vi "Trans-RT.vi"() -> ()   [LabVIEW 2016]
uses:
  <vilib>/rvi/interface/nirviOpenFPGA/nirviOpenFPGA.xnode
  <vilib>/rvi/interface/nirviReadWriteControl/nirviReadWriteControl.xnode
  <vilib>/functionblocks/FB Core/FB Core.xnode
  <vilib>/functionblocks/Control/PID/PID.vi
  <vilib>/functionblocks/NI_FunctionBlock Libraries.lvlib
  Common-Control/Beamline sections/Transmission/Trans-FPGA.vi
  NiFpgaLv.dll
  <vilib>/Utility/error.llb/Error Cluster From Error Code.vi
  <vilib>/rvi/errors/niLvFpgaAdjustHostInterfaceError.vi
  <vilib>/functionblocks/FB Property/FB Overlay DBL.ctl
  Controls/GV states.ctl
  Controls/Faraday cup states.ctl
  <vilib>/NI_Real-Time Target Support.lvlib
  FPGA Bitfiles/PRIMEControl2017_FPGATarget4_Trans-FPGA_w9NSCwWceHg.lvbitx
  <vilib>/FPGAPlugInAG/cRIO-9067/niLvFpga_Open_cRIO-9067.vi
  GP307 cluster.ctl
panel:
  in  "Tab Control":T1(tab)
  out "Steerer X+":dbl
  out "Steerer X-":dbl
  out "Steerer Y+":dbl
  out "Steerer Y-":dbl
  out "ExB +":dbl
  out "ExB -":dbl
  out "X+ V":fxp<+/-,26,5> format="%.23g"
  out "X+ I":fxp<+/-,26,5> format="%_4g"
  out "X- V":fxp<+/-,26,5> format="%_4g"
  out "X- I":fxp<+/-,26,5> format="%_4g"
  out "Y+ V":fxp<+/-,26,5> format="%_4g"
  out "Y+ I":fxp<+/-,26,5> format="%_4g"
  out "Y- V":fxp<+/-,26,5> format="%_4g"
  out "Y- I":fxp<+/-,26,5> format="%_4g"
  out "ExB+ V":fxp<+/-,26,5> format="%_4g"
  out "ExB+ I":fxp<+/-,26,5> format="%_4g"
  out "ExB- V":fxp<+/-,26,5> format="%_4g"
  out "ExB- I":fxp<+/-,26,5> format="%_4g"
  out "ExB- HV Enable":bool
  out "ExB+ HV Enable":bool
  out "X-steerer+ HV Enable":bool
  out "X-steerer- HV Enable":bool
  out "Y-steerer+ HV Enable":bool
  out "Y-steerer- HV Enable":bool
  in  "derivative time (Td, min) -analyzer":dbl=0.05
  in  "integral time (Ti, min) -analyzer":dbl=0.01
  in  "proportional gain (Kc) -analyzer":dbl=25.0
  out "Analyzer mag command string":string
  out "analyzer field read":dbl
  out "Analyzer mag command":u8[](array[numeric])
  out "Analyzer mag field read":u8[](array[numeric])
  out "Analyzer mag field set":dbl
  in  "output high - analyzer":dbl=300.0
  in  "output low - analyzer":dbl
  out "Switch mag field set":dbl
  out "Switch mag field read":u8[](array[numeric])
  out "switch mag field read":dbl
  out "Switch mag command":u8[](array[numeric])
  in  "derivative time (Td, min) - switch":dbl=0.01
  in  "integral time (Ti, min) - switch":dbl=0.01
  in  "proportional gain (Kc) - switch":dbl=10.0
  out "Switch mag command string":string
  in  "output high - switch":dbl=250.0
  in  "output low - switch":dbl
  out "ExB mag command":u8[](array[numeric])
  out "EXB":dbl
  out "ExB mag command string":string
  in  "Ion gauge cluster control":T2
  out "Analyze image vac gauge cluster":T3
  out "Switch object vac gauge cluster":T3
  out "Convectron 4":u8[](array[numeric])
  out "Ion gauge 4":u8[](array[numeric])
  out "Convectron 3":u8[](array[numeric])
  out "Ion gauge 3":u8[](array[numeric])
  out "Convectron 2":u8[](array[numeric])
  out "Ion gauge 2":u8[](array[numeric])
  out "Convectron 1":u8[](array[numeric])
  out "Ion gauge 1":u8[](array[numeric])
  out "Analzyer Image FC Actuator":bool
  out "Beamline GV Actuator":bool
  out "Turbo 1 GV Actuator":bool
  out "Turbo 2 GV Actuator":bool
  out "Switch Object Vac Interlock":bool
  out "Analyzer Image Vac Interlock":bool
  out "Turbo 1 GV status 2":T4
  out "Turbo 1 GV status":T5
  out "Turbo 2 GV status 2":T4
  out "Turbo 2 GV status":T5
  out "Beamline GV status 2":T4
  out "Beamline GV status":T5
  out "Analyzer Image FC Position":cluster{"IN sensor":bool, "OUT sensor":bool}
  out "Analyzer Image FC Status":T6
  out "Readback loop error":errorcluster
  out "Vacuum loop error":errorcluster
  out "Control Loop error":errorcluster
  out "ExB error":errorcluster
  out "Switch Magnet error":errorcluster
  out "Analyzer Magnet error":errorcluster
  out "Error Reporter":errorcluster
  out "Actuator Sensor loop error":errorcluster
  out "Interlock loop error":errorcluster
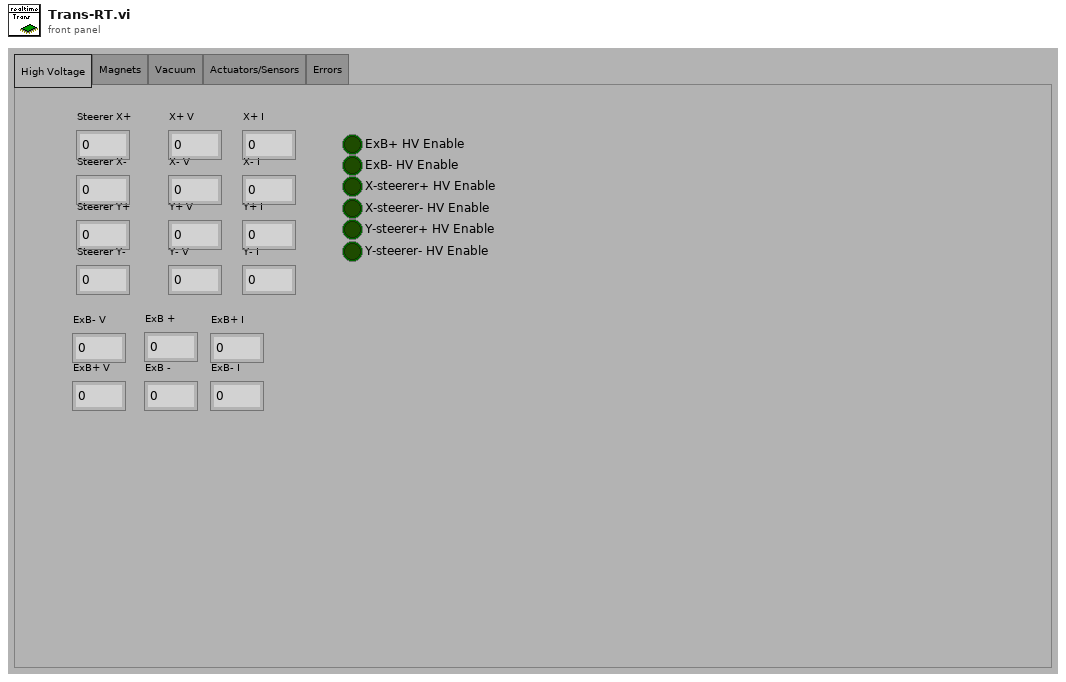
[diagram p1: front panel]
types:
  T1 = enum32{"High Voltage", "Magnets", "Vacuum", "Actuators/Sensors", "Errors"}
  T2 = typedef "GP307 cluster.ctl" = cluster{"Ion gauge 1":string, "Convectron  Gauge 1 ":string, "Ion Gauge 2":string, "Convectrom Gauge 2":string}
  T3 = cluster{"Ion gauge 1":string, "Convectron  Gauge 1 ":string, "Ion Gauge 2":string, "Convectrom Gauge 2":string}
  T4 = typedef "GV states.ctl" = enum16{"status unclear", "closed", "open"}
  T5 = cluster{"OPEN sensor":bool, "Closed sensor":bool}
  T6 = typedef "Faraday cup states.ctl" = enum16{"FC status unclear", "FC in", "FC out"}
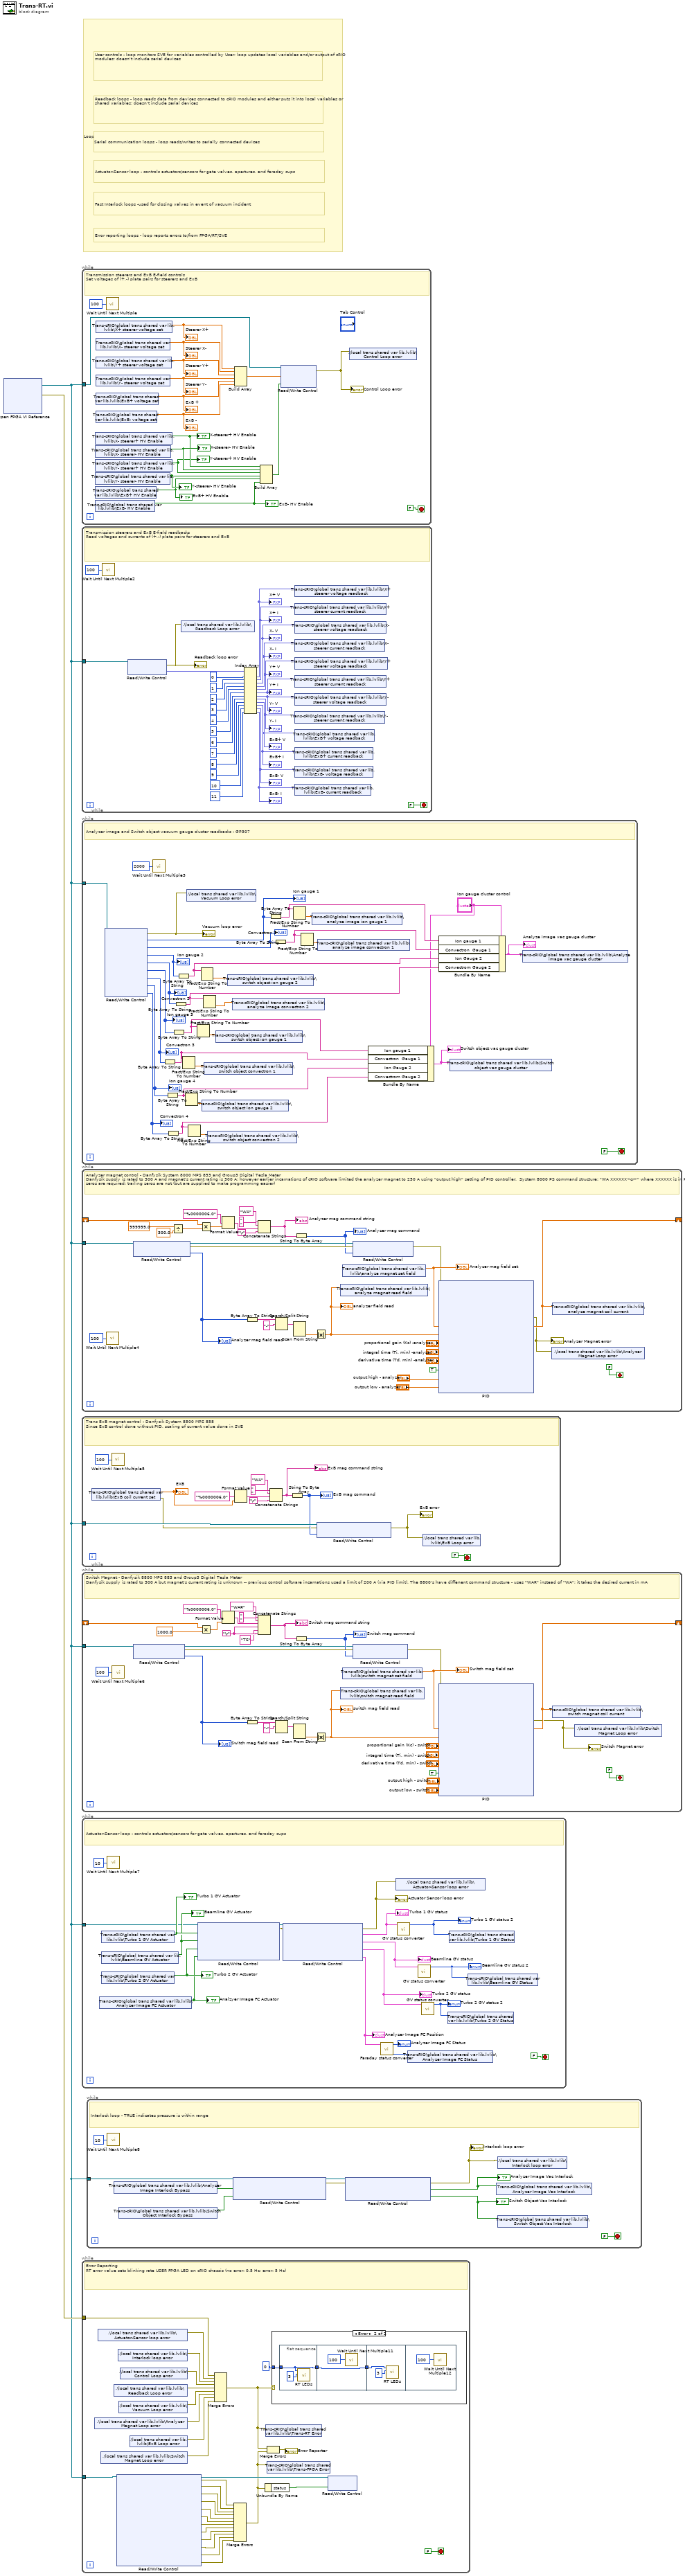
[diagram p0: block diagram]
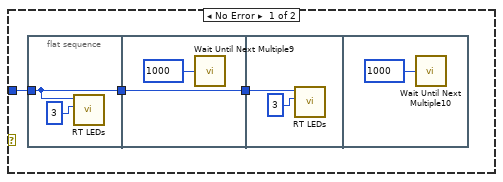
[diagram p2: hidden frame]
diagram:
  # "Serial communication loops - loop reads/writes to serially connected devices"
  # "Actuator-Sensor loop - controls actuators/sensors for gate valves, apertures, and faraday cups"
  # "Fast Interlock loops -used for closing valves in event of vacuum incident"
  # "Error reporting loops - loop reports errors to/from FPGA/RT/SVE"
  # "Readback loops - loop reads data from devices connected to cRIO modules and either puts it into local variables or shared variables; doesn't include serial devices"
  # "User controls - loop monitors SVE for variables controlled by User; loop updates local variables and/or output of cRIO modules; doesn't include serial devices"
  # "Loop legend - loops are color coded by responsibility"
  n1 = xnode "Open FPGA VI Reference"() -> ("FPGA VI Reference Out"=w1:refnum<k20>, "error out"=w2:errorcluster)  [unwired: 2 in]
  n2 = while {
    tunnel: w1 -> [w11]
    stop <- FALSE stop-if-true
    # "Transmission steerers and ExB E-field controls\nSet voltages of (+,-) plate pairs for steerers and ExB"
    n3 = shared-variable "Trans-cRIO\\global trans shared var lib.lvlib\\X- steerer+ HV Enable"() -> (w6:bool)  [unwired: 1 in, 1 out]
    "X-steerer+ HV Enable" <- w6
    n4 = shared-variable "Trans-cRIO\\global trans shared var lib.lvlib\\X- steerer- HV Enable"() -> (w7:bool)  [unwired: 1 in, 1 out]
    "X-steerer- HV Enable" <- w7
    n5 = shared-variable "Trans-cRIO\\global trans shared var lib.lvlib\\Y- steerer+ HV Enable"() -> (w4:bool)  [unwired: 1 in, 1 out]
    "Y-steerer+ HV Enable" <- w4
    n6 = shared-variable "Trans-cRIO\\global trans shared var lib.lvlib\\Y- steerer- HV Enable"() -> (w8:bool)  [unwired: 1 in, 1 out]
    "Y-steerer- HV Enable" <- w8
    n7 = shared-variable "Trans-cRIO\\global trans shared var lib.lvlib\\ExB+ HV Enable"() -> (w5:bool)  [unwired: 1 in, 1 out]
    "ExB+ HV Enable" <- w5
    n8 = shared-variable "Trans-cRIO\\global trans shared var lib.lvlib\\ExB- HV Enable"() -> (w9:bool)  [unwired: 1 in, 1 out]
    "ExB- HV Enable" <- w9
    n9 = shared-variable "Trans-cRIO\\global trans shared var lib.lvlib\\X+ steerer voltage set"() -> (w13:dbl)  [unwired: 1 in, 1 out]
    "Steerer X+" <- w13
    n10 = shared-variable "Trans-cRIO\\global trans shared var lib.lvlib\\X- steerer voltage set"() -> (w14:dbl)  [unwired: 1 in, 1 out]
    "Steerer X-" <- w14
    n11 = shared-variable "Trans-cRIO\\global trans shared var lib.lvlib\\Y+ steerer voltage set"() -> (w15:dbl)  [unwired: 1 in, 1 out]
    "Steerer Y+" <- w15
    n12 = shared-variable "Trans-cRIO\\global trans shared var lib.lvlib\\Y- steerer voltage set"() -> (w16:dbl)  [unwired: 1 in, 1 out]
    "Steerer Y-" <- w16
    n13 = shared-variable "Trans-cRIO\\global trans shared var lib.lvlib\\ExB+ voltage set"() -> (w17:dbl)  [unwired: 1 in, 1 out]
    "ExB +" <- w17
    n14 = shared-variable "Trans-cRIO\\global trans shared var lib.lvlib\\ExB- voltage set"() -> (w18:dbl)  [unwired: 1 in, 1 out]
    "ExB -" <- w18
    n15 = call "Wait Until Next Multiple"("Count(mSec)"=u32 100 ("millisecond multiple")) -> ()  [unwired: 1 out]
    n16 = Build Array(w13, w14, w15, w16, w17, w18) -> (w20:dbl[])
    n17 = Build Array(w6, w7, w4, w8, w5, w9) -> (w10:bool[])
    n18 = xnode "Read/Write Control"("FPGA VI Reference In"=w11, "HV Set"=w20, "HV Enable"=w10) -> ("error out"=w12:errorcluster)  [unwired: 1 in, 1 out]
    "Control Loop error" <- w12
    n19 = shared-variable ".\\local trans shared var lib.lvlib\\Control Loop error"(w12) -> ()  [unwired: 1 in, 1 out]
  }
  n20 = while {
    tunnel: w1 -> [w23]
    stop <- FALSE stop-if-true
    # "Transmission steerers and ExB E-field readbacks\nRead voltages and currents of (+,-) plate pairs for steerers and ExB"
    n21 = call "Wait Until Next Multiple2"("Count(mSec)"=u32 100 ("millisecond multiple")) -> ()  [unwired: 1 out]
    n22 = xnode "Read/Write Control"("FPGA VI Reference In"=w23) -> ("error out"=w22:errorcluster, "HV monitor"=w49:fxp<+/-,26,5>[])  [unwired: 1 in, 1 out]
    "Readback loop error" <- w22
    n23 = shared-variable ".\\local trans shared var lib.lvlib\\Readback Loop error"(w22) -> ()  [unwired: 1 in, 1 out]
    n24 = Index Array(array=w49, index #1=0 ("index"), index #2=1 ("index"), index #3=2 ("index"), index #4=3 ("index"), index #5=4 ("index"), index #6=5 ("index"), index #7=6 ("index"), index #8=7 ("index"), index #9=8 ("index"), index #10=9 ("index"), index #11=10 ("index"), index #12=11 ("index")) -> (element #1=w38:fxp<+/-,26,5>, element #2=w40:fxp<+/-,26,5>, element #3=w39:fxp<+/-,26,5>, element #4=w37:fxp<+/-,26,5>, element #5=w41:fxp<+/-,26,5>, element #6=w43:fxp<+/-,26,5>, element #7=w42:fxp<+/-,26,5>, element #8=w44:fxp<+/-,26,5>, element #9=w45:fxp<+/-,26,5>, element #10=w47:fxp<+/-,26,5>, element #11=w46:fxp<+/-,26,5>, element #12=w48:fxp<+/-,26,5>)
    "X+ V" <- w38
    "X+ I" <- w40
    "X- V" <- w39
    "X- I" <- w37
    "Y+ V" <- w41
    "Y+ I" <- w43
    "Y- V" <- w42
    "Y- I" <- w44
    "ExB+ V" <- w45
    "ExB+ I" <- w47
    "ExB- V" <- w46
    "ExB- I" <- w48
    n25 = shared-variable "Trans-cRIO\\global trans shared var lib.lvlib\\X+ steerer voltage readback"(w38) -> ()  [unwired: 1 in, 1 out]
    n26 = shared-variable "Trans-cRIO\\global trans shared var lib.lvlib\\X+ steerer current readback"(w40) -> ()  [unwired: 1 in, 1 out]
    n27 = shared-variable "Trans-cRIO\\global trans shared var lib.lvlib\\X- steerer voltage readback"(w39) -> ()  [unwired: 1 in, 1 out]
    n28 = shared-variable "Trans-cRIO\\global trans shared var lib.lvlib\\X- steerer current readback"(w37) -> ()  [unwired: 1 in, 1 out]
    n29 = shared-variable "Trans-cRIO\\global trans shared var lib.lvlib\\Y+ steerer voltage readback"(w41) -> ()  [unwired: 1 in, 1 out]
    n30 = shared-variable "Trans-cRIO\\global trans shared var lib.lvlib\\Y+ steerer current readback"(w43) -> ()  [unwired: 1 in, 1 out]
    n31 = shared-variable "Trans-cRIO\\global trans shared var lib.lvlib\\Y- steerer voltage readback"(w42) -> ()  [unwired: 1 in, 1 out]
    n32 = shared-variable "Trans-cRIO\\global trans shared var lib.lvlib\\Y- steerer current readback"(w44) -> ()  [unwired: 1 in, 1 out]
    n33 = shared-variable "Trans-cRIO\\global trans shared var lib.lvlib\\ExB+ voltage readback"(w45) -> ()  [unwired: 1 in, 1 out]
    n34 = shared-variable "Trans-cRIO\\global trans shared var lib.lvlib\\ExB+ current readback"(w47) -> ()  [unwired: 1 in, 1 out]
    n35 = shared-variable "Trans-cRIO\\global trans shared var lib.lvlib\\ExB- voltage readback"(w46) -> ()  [unwired: 1 in, 1 out]
    n36 = shared-variable "Trans-cRIO\\global trans shared var lib.lvlib\\ExB- current readback"(w48) -> ()  [unwired: 1 in, 1 out]
  }
  n37 = while {
    tunnel: w1 -> [w56]
    stop <- FALSE stop-if-true
    # "Analyzer image and Switch object vacuum gauge cluster readbacks - GP307"
    n38 = xnode "Read/Write Control"("FPGA VI Reference In"=w56) -> ("error out"=w55:errorcluster, "Ion gauge 1"=w77:u8[], "Convectron 1"=w78:u8[], "Ion gauge 2"=w79:u8[], "Convectron 2"=w80:u8[], "Ion gauge 3"=w75:u8[], "Convectron 3"=w74:u8[], "Ion gauge 4"=w53:u8[], "Convectron 4"=w52:u8[])  [unwired: 1 in, 1 out]
    "Vacuum loop error" <- w55
    "Ion gauge 1" <- w77
    "Convectron 1" <- w78
    "Ion gauge 2" <- w79
    "Convectron 2" <- w80
    "Ion gauge 3" <- w75
    "Convectron 3" <- w74
    "Ion gauge 4" <- w53
    "Convectron 4" <- w52
    n39 = call "Wait Until Next Multiple3"("Count(mSec)"=u32 2000 ("millisecond multiple")) -> ()  [unwired: 1 out]
    n40 = Byte Array To String(unsigned byte array=w74) -> (string=w71:string)
    n41 = Byte Array To String(unsigned byte array=w53) -> (string=w70:string)
    n42 = Byte Array To String(unsigned byte array=w52) -> (string=w69:string)
    n43 = Byte Array To String(unsigned byte array=w75) -> (string=w72:string)
    n44 = Byte Array To String(unsigned byte array=w80) -> (string=w62:string)
    n45 = Byte Array To String(unsigned byte array=w79) -> (string=w61:string)
    n46 = Fract/Exp String To Number(string=w71) -> (number=w67:dbl)  [unwired: 3 in, 1 out]
    n47 = Fract/Exp String To Number(string=w70) -> (number=w66:dbl)  [unwired: 3 in, 1 out]
    n48 = shared-variable ".\\local trans shared var lib.lvlib\\Vacuum Loop error"(w55) -> ()  [unwired: 1 in, 1 out]
    n49 = Fract/Exp String To Number(string=w69) -> (number=w65:dbl)  [unwired: 3 in, 1 out]
    n50 = Fract/Exp String To Number(string=w72) -> (number=w68:dbl)  [unwired: 3 in, 1 out]
    n51 = Fract/Exp String To Number(string=w61) -> (number=w59:dbl)  [unwired: 3 in, 1 out]
    n52 = shared-variable "Trans-cRIO\\global trans shared var lib.lvlib\\switch object ion gauge 2"(w66) -> ()  [unwired: 1 in, 1 out]
    n53 = Fract/Exp String To Number(string=w62) -> (number=w57:dbl)  [unwired: 3 in, 1 out]
    n54 = shared-variable "Trans-cRIO\\global trans shared var lib.lvlib\\switch object convectron 1"(w67) -> ()  [unwired: 1 in, 1 out]
    n55 = shared-variable "Trans-cRIO\\global trans shared var lib.lvlib\\switch object convectron 2"(w65) -> ()  [unwired: 1 in, 1 out]
    n56 = shared-variable "Trans-cRIO\\global trans shared var lib.lvlib\\switch object ion gauge 1"(w68) -> ()  [unwired: 1 in, 1 out]
    n57 = shared-variable "Trans-cRIO\\global trans shared var lib.lvlib\\switch object ion gauge 2"(w59) -> ()  [unwired: 1 in, 1 out]
    n58 = shared-variable "Trans-cRIO\\global trans shared var lib.lvlib\\analyze image convectron 2"(w57) -> ()  [unwired: 1 in, 1 out]
    n59 = Byte Array To String(unsigned byte array=w77) -> (string=w64:string)
    n60 = Byte Array To String(unsigned byte array=w78) -> (string=w63:string)
    n61 = Fract/Exp String To Number(string=w64) -> (number=w60:dbl)  [unwired: 3 in, 1 out]
    n62 = Fract/Exp String To Number(string=w63) -> (number=w58:dbl)  [unwired: 3 in, 1 out]
    n63 = shared-variable "Trans-cRIO\\global trans shared var lib.lvlib\\analyze image ion gauge 1"(w60) -> ()  [unwired: 1 in, 1 out]
    n64 = shared-variable "Trans-cRIO\\global trans shared var lib.lvlib\\analyze image convectron 1"(w58) -> ()  [unwired: 1 in, 1 out]
    n65 = Bundle By Name(cluster="Ion gauge cluster control", "Ion gauge 1"=w72, "Convectron  Gauge 1"=w71, "Ion Gauge 2"=w70, "Convectrom Gauge 2"=w69) -> (w73:T2)
    "Switch object vac gauge cluster" <- w73
    n66 = Bundle By Name(cluster="Ion gauge cluster control", "Ion gauge 1"=w64, "Convectron  Gauge 1"=w63, "Ion Gauge 2"=w61, "Convectrom Gauge 2"=w62) -> (w54:T2)
    "Analyze image vac gauge cluster" <- w54
    n67 = shared-variable "Trans-cRIO\\global trans shared var lib.lvlib\\Switch object vac gauge cluster"(w73) -> ()  [unwired: 1 in, 1 out]
    n68 = shared-variable "Trans-cRIO\\global trans shared var lib.lvlib\\Analyze image vac gauge cluster"(w54) -> ()  [unwired: 1 in, 1 out]
  }
  n69 = while {
    shift-right: [w99] -> _
    shift-left: _ -> [w90]
    tunnel: w1 -> [w94]
    stop <- FALSE stop-if-true
    # "Analyzer magnet control - Danfysik System 8000 MPS 853 and Group3 Digital Tesla Meter\nDanfysik supply is rated to 300 A and magnet's current rating is 300 A; however earlier incarnations of cRIO software limited the analyzer magnet to 250 A using \"output high\" setting of PID controller.  System 8000 PS command structure: \"WA XXXXXX<cr>\" where XXXXXX is in PPM of full current. Leading zeros are required; trailing zeros are not (but are supplied to make programming easier)"
    n70 = call "Wait Until Next Multiple4"("Count(mSec)"=u32 100 ("millisecond multiple")) -> ()  [unwired: 1 out]
    n71 = xnode "Read/Write Control"("FPGA VI Reference In"=w94) -> ("FPGA VI Reference Out"=w86:refnum<k20>, "error out"=w93:errorcluster, "analyzer mag field"=w89:u8[])  [unwired: 1 in]
    "Analyzer mag field read" <- w89
    n72 = Divide(x=999999.0, y=300.0) -> (x/y=w106:dbl)
    n73 = Multiply(x=w90, y=w106) -> (x*y=w108:dbl)
    n74 = Format Value(format string="%0000006.0", value (0)=w108) -> (output string=w111:string)  [unwired: 1 out]
    n75 = Byte Array To String(unsigned byte array=w89) -> (string=w101:string)
    n76 = Concatenate Strings("WA", " ", w111, "\r") -> (w112:string)
    "Analyzer mag command string" <- w112
    n77 = Search/Split String(string=w101, search string/char (-)="-") -> (match + rest of string=w91:string)  [unwired: 3 out]
    n78 = Scan From String(input string=w91) -> (output 1=w100:dbl)  [unwired: 3 in, 4 out]
    n79 = String To Byte Array(string=w112) -> (unsigned byte array=w92:u8[])
    "Analyzer mag command" <- w92
    n80 = Absolute Value(x=w100) -> (abs(x)=w87:dbl)
    "analyzer field read" <- w87
    n81 = shared-variable "Trans-cRIO\\global trans shared var lib.lvlib\\analyze magnet read field"(w87) -> ()  [unwired: 1 in, 1 out]
    n82 = shared-variable "Trans-cRIO\\global trans shared var lib.lvlib\\analyze magnet set field"() -> (w88:dbl)  [unwired: 1 in, 1 out]
    "Analyzer mag field set" <- w88
    n83 = xnode "Read/Write Control"("FPGA VI Reference In"=w86, "error in"=w93, "analyzer mag ps set"=w92) -> ("error out"=w85:errorcluster)  [unwired: 1 out]
    n84 = xnode "PID"("error in"=w85, "setpoint"=w88, "process variable"=w87, "proportional gain (Kc)"="proportional gain (Kc) -analyzer", "integral time (Ti, min)"="integral time (Ti, min) -analyzer", "derivative time (Td, min)"="derivative time (Td, min) -analyzer", "auto? (T)"=TRUE, "output high"="output high - analyzer", "output low"="output low - analyzer") -> ("error out"=w84:errorcluster, "output"=w99:dbl)
    "Analyzer Magnet error" <- w84
    n85 = shared-variable ".\\local trans shared var lib.lvlib\\Analyzer Magnet Loop error"(w84) -> ()  [unwired: 1 in, 1 out]
    n86 = shared-variable "Trans-cRIO\\global trans shared var lib.lvlib\\analyze magnet coil current"(w99) -> ()  [unwired: 1 in, 1 out]
  }
  n87 = while {
    tunnel: w1 -> [w185]
    stop <- FALSE stop-if-true
    # "Trans ExB magnet control - Danfysik System 8500 MPS 858\nSince ExB control done without PID, scaling of current value done in SVE"
    n88 = shared-variable "Trans-cRIO\\global trans shared var lib.lvlib\\ExB coil current set"() -> (w182:dbl, error out=w181:errorcluster)  [unwired: 1 in]
    "EXB" <- w182
    n89 = call "Wait Until Next Multiple5"("Count(mSec)"=u32 100 ("millisecond multiple")) -> ()  [unwired: 1 out]
    n90 = Format Value(format string="%0000006.0", value (0)=w182) -> (output string=w189:string)  [unwired: 1 out]
    n91 = Concatenate Strings("WA", " ", w189, "\r") -> (w186:string)
    "ExB mag command string" <- w186
    n92 = String To Byte Array(string=w186) -> (unsigned byte array=w183:u8[])
    "ExB mag command" <- w183
    n93 = xnode "Read/Write Control"("FPGA VI Reference In"=w185, "error in"=w181, "trans ExB mag ps set"=w183) -> ("error out"=w184:errorcluster)  [unwired: 1 out]
    "ExB error" <- w184
    n94 = shared-variable ".\\local trans shared var lib.lvlib\\ExB Loop error"(w184) -> ()  [unwired: 1 in, 1 out]
  }
  n95 = while {
    shift-right: [w214] -> _
    shift-left: _ -> [w205]
    tunnel: w1 -> [w209]
    stop <- FALSE stop-if-true
    w197 = "\r"
    # "Switch Magnet - Danfysik 8800 MPS 883 and Group3 Digital Tesla Meter\nDanfysik supply is rated to 300 A but magnet's current rating is unknown -- previous control software incarnations used a limit of 200 A (via PID limit). The 8800's have diffenent command structure - uses \"WAR\" instead of \"WA\"; it takes the desired current in mA"
    n96 = call "Wait Until Next Multiple6"("Count(mSec)"=u32 100 ("millisecond multiple")) -> ()  [unwired: 1 out]
    n97 = xnode "Read/Write Control"("FPGA VI Reference In"=w209) -> ("FPGA VI Reference Out"=w201:refnum<k20>, "error out"=w208:errorcluster, "switch mag field"=w204:u8[])  [unwired: 1 in]
    "Switch mag field read" <- w204
    n98 = Multiply(x=w205, y=1000.0) -> (x*y=w220:dbl)
    n99 = Format Value(format string="%0000006.0", value (0)=w220) -> (output string=w223:string)  [unwired: 1 out]
    n100 = Byte Array To String(unsigned byte array=w204) -> (string=w216:string)
    n101 = Concatenate Strings("WAR", " ", w223, w197, "TS" ("string"), w197) -> (w224:string)
    "Switch mag command string" <- w224
    n102 = Search/Split String(string=w216, search string/char (-)="-") -> (match + rest of string=w206:string)  [unwired: 3 out]
    n103 = Scan From String(input string=w206) -> (output 1=w215:dbl)  [unwired: 3 in, 4 out]
    n104 = String To Byte Array(string=w224) -> (unsigned byte array=w207:u8[])
    "Switch mag command" <- w207
    n105 = Absolute Value(x=w215) -> (abs(x)=w202:dbl)
    "switch mag field read" <- w202
    n106 = shared-variable "Trans-cRIO\\global trans shared var lib.lvlib\\switch magnet read field"(w202) -> ()  [unwired: 1 in, 1 out]
    n107 = shared-variable "Trans-cRIO\\global trans shared var lib.lvlib\\switch magnet set field"() -> (w203:dbl)  [unwired: 1 in, 1 out]
    "Switch mag field set" <- w203
    n108 = xnode "Read/Write Control"("FPGA VI Reference In"=w201, "error in"=w208, "switch mag ps set"=w207) -> ("error out"=w200:errorcluster)  [unwired: 1 out]
    n109 = xnode "PID"("error in"=w200, "setpoint"=w203, "process variable"=w202, "proportional gain (Kc)"="proportional gain (Kc) - switch", "integral time (Ti, min)"="integral time (Ti, min) - switch", "derivative time (Td, min)"="derivative time (Td, min) - switch", "auto? (T)"=TRUE, "output high"="output high - switch", "output low"="output low - switch") -> ("error out"=w199:errorcluster, "output"=w214:dbl)
    "Switch Magnet error" <- w199
    n110 = shared-variable "Trans-cRIO\\global trans shared var lib.lvlib\\switch magnet coil current"(w214) -> ()  [unwired: 1 in, 1 out]
    n111 = shared-variable ".\\local trans shared var lib.lvlib\\Switch Magnet Loop error"(w199) -> ()  [unwired: 1 in, 1 out]
  }
  n112 = while {
    tunnel: w1 -> [w301]
    stop <- FALSE stop-if-true
    # "Actuator-Sensor loop - controls actuators/sensors for gate valves, apertures, and faraday cups"
    n113 = shared-variable "Trans-cRIO\\global trans shared var lib.lvlib\\Analyzer Image FC Actuator"() -> (w294:bool)  [unwired: 1 in, 1 out]
    "Analzyer Image FC Actuator" <- w294
    n114 = shared-variable "Trans-cRIO\\global trans shared var lib.lvlib\\Turbo 1 GV Actuator"() -> (w304:bool)  [unwired: 1 in, 1 out]
    "Turbo 1 GV Actuator" <- w304
    n115 = shared-variable "Trans-cRIO\\global trans shared var lib.lvlib\\Beamline GV Actuator"() -> (w303:bool)  [unwired: 1 in, 1 out]
    "Beamline GV Actuator" <- w303
    n116 = shared-variable "Trans-cRIO\\global trans shared var lib.lvlib\\Turbo 2 GV Actuator"() -> (w297:bool)  [unwired: 1 in, 1 out]
    "Turbo 2 GV Actuator" <- w297
    n117 = call "Wait Until Next Multiple7"("Count(mSec)"=u32 10 ("millisecond multiple")) -> ()  [unwired: 1 out]
    n118 = xnode "Read/Write Control"("FPGA VI Reference In"=w301, "Turbo 1 GV Actuator"=w304, "Beamline GV Actuator"=w303, "Turbo 2 GV Actuator"=w297, "Analzyer Image FC Actuator"=w294) -> ("FPGA VI Reference Out"=w307:refnum<k20>, "error out"=w306:errorcluster)  [unwired: 1 in]
    n119 = xnode "Read/Write Control"("FPGA VI Reference In"=w307, "error in"=w306) -> ("error out"=w305:errorcluster, "Turbo 1 GV Status"=w300:T5, "Turbo 2 GV Status"=w299:T5, "Beamline GV Status"=w298:T5, "Analzyer Image FC Position"=w292:cluster{"IN sensor":bool, "OUT sensor":bool})  [unwired: 1 out]
    "Actuator Sensor loop error" <- w305
    "Beamline GV status" <- w299
    "Turbo 2 GV status" <- w298
    "Turbo 1 GV status" <- w300
    "Analyzer Image FC Position" <- w292
    n120 = call "Faraday status converter.vi"("FC Position"=w292) -> ("FC Status"=w293:T6)  [unwired: 10 in]
    "Analyzer Image FC Status" <- w293
    n121 = shared-variable ".\\local trans shared var lib.lvlib\\Actuator-Sensor loop error"(w305) -> ()  [unwired: 1 in, 1 out]
    n122 = call "GV status converter.vi"("Gate Valve"=w300) -> ("GV Status"=w302:T4)  [unwired: 10 in]
    "Turbo 1 GV status 2" <- w302
    n123 = shared-variable "Trans-cRIO\\global trans shared var lib.lvlib\\Analyzer Image FC Status"(w293) -> ()  [unwired: 1 in, 1 out]
    n124 = call "GV status converter.vi"("Gate Valve"=w299) -> ("GV Status"=w296:T4)  [unwired: 10 in]
    "Beamline GV status 2" <- w296
    n125 = call "GV status converter.vi"("Gate Valve"=w298) -> ("GV Status"=w295:T4)  [unwired: 10 in]
    "Turbo 2 GV status 2" <- w295
    n126 = shared-variable "Trans-cRIO\\global trans shared var lib.lvlib\\Turbo 2 GV Status"(w295) -> ()  [unwired: 1 in, 1 out]
    n127 = shared-variable "Trans-cRIO\\global trans shared var lib.lvlib\\Turbo 1 GV Status"(w302) -> ()  [unwired: 1 in, 1 out]
    n128 = shared-variable "Trans-cRIO\\global trans shared var lib.lvlib\\Beamline GV Status"(w296) -> ()  [unwired: 1 in, 1 out]
  }
  n129 = while {
    tunnel: w1 -> [w336]
    tunnel: w2 -> [w313]
    stop <- FALSE stop-if-true
    # "Error Reporting\nRT error value sets blinking rate USER FPGA LED on cRIO chassis (no error: 0.5 Hz; error: 5 Hz)"
    n130 = shared-variable ".\\local trans shared var lib.lvlib\\Analyzer Magnet Loop error"() -> (w319:errorcluster)  [unwired: 1 in, 1 out]
    n131 = shared-variable ".\\local trans shared var lib.lvlib\\Actuator-Sensor loop error"() -> (w314:errorcluster)  [unwired: 1 in, 1 out]
    n132 = shared-variable ".\\local trans shared var lib.lvlib\\Switch Magnet Loop error"() -> (w321:errorcluster)  [unwired: 1 in, 1 out]
    n133 = shared-variable ".\\local trans shared var lib.lvlib\\Readback Loop error"() -> (w317:errorcluster)  [unwired: 1 in, 1 out]
    n134 = xnode "Read/Write Control"("FPGA VI Reference In"=w336) -> ("FPGA VI Reference Out"=w335:refnum<k20>, "error out"=w322:errorcluster, "9205 error"=w334:errorcluster, "9264 error"=w333:errorcluster, "Analyzer PS error"=w332:errorcluster, "ExB PS error"=w331:errorcluster, "Switch PS error"=w330:errorcluster, "Analyzer Hall Probe error"=w329:errorcluster, "Switch Hall Probe error"=w328:errorcluster, "Analyze Image Vacuum Error"=w327:errorcluster, "Switch Object Vacuum Error"=w326:errorcluster, "GV Interlock loop error"=w324:errorcluster, "Actuator-Sensor Loop error"=w323:errorcluster)  [unwired: 1 in]
    n135 = shared-variable ".\\local trans shared var lib.lvlib\\Interlock loop error"() -> (w315:errorcluster)  [unwired: 1 in, 1 out]
    n136 = shared-variable ".\\local trans shared var lib.lvlib\\Vacuum Loop error"() -> (w318:errorcluster)  [unwired: 1 in, 1 out]
    n137 = shared-variable ".\\local trans shared var lib.lvlib\\Control Loop error"() -> (w316:errorcluster)  [unwired: 1 in, 1 out]
    n138 = shared-variable ".\\local trans shared var lib.lvlib\\ExB Loop error"() -> (w320:errorcluster)  [unwired: 1 in, 1 out]
    n139 = Merge Errors(w313, w314, w315, w316, w317, w318, w319, w320, w321) -> (w309:errorcluster)
    n140 = Merge Errors(w322, w334, w333, w332, w331, w330, w329, w328, w327, w326, w324, w323) -> (w312:errorcluster)
    n141 = Unbundle By Name(w312) -> ("status"=w337:bool)
    n142 = shared-variable "Trans-cRIO\\global trans shared var lib.lvlib\\Trans-RT Error"(w309) -> ()  [unwired: 1 in, 1 out]
    n143 = Merge Errors(w309, w312) -> (→"Error Reporter":errorcluster)
    n144 = shared-variable "Trans-cRIO\\global trans shared var lib.lvlib\\Trans-FPGA Error"(w312) -> ()  [unwired: 1 in, 1 out]
    n145 = case shown="Error" w309 {
      tunnel: 0 -> [w340 w348]
      frame No Error {
        n146 = flat-sequence {
          tunnel: w340 -> [w341]
          tunnel: [w341] -> w338
          tunnel: [w343] -> w339
          tunnel: w338 -> [w343]
          tunnel: w339 -> [w345]
          frame #0 {
            n147 = call <vilib>:"RT LEDs.vi"("State"=3, "LED Num"=w341) -> ()  [unwired: 4 in, 2 out]
          }
          frame #1 {
            n148 = call "Wait Until Next Multiple9"("Count(mSec)"=u16 1000) -> ()  [unwired: 1 out]
          }
          frame #2 {
            n149 = call <vilib>:"RT LEDs.vi"("State"=3, "LED Num"=w345) -> ()  [unwired: 4 in, 2 out]
          }
          frame #3 {
            n150 = call "Wait Until Next Multiple10"("Count(mSec)"=u16 1000) -> ()  [unwired: 1 out]
          }
        }
      }
      frame Error {
        n151 = flat-sequence {
          tunnel: [w351] -> w350
          tunnel: w348 -> [w351]
          tunnel: w350 -> [w353]
          tunnel: [w353] -> w349
          tunnel: w349 -> [w355]
          frame #0 {
            n152 = call <vilib>:"RT LEDs.vi"("State"=3, "LED Num"=w351) -> ()  [unwired: 4 in, 2 out]
          }
          frame #1 {
            n153 = call "Wait Until Next Multiple11"("Count(mSec)"=u16 100) -> ()  [unwired: 1 out]
          }
          frame #2 {
            n154 = call <vilib>:"RT LEDs.vi"("State"=3, "LED Num"=w355) -> ()  [unwired: 4 in, 2 out]
          }
          frame #3 {
            n155 = call "Wait Until Next Multiple12"("Count(mSec)"=u16 100) -> ()  [unwired: 1 out]
          }
        }
      }
    }
    n156 = xnode "Read/Write Control"("FPGA VI Reference In"=w335, "RT error"=w337) -> ()  [unwired: 1 in, 2 out]
  }
  n157 = while {
    tunnel: w1 -> [w363]
    stop <- FALSE stop-if-true
    # "Interlock loop - TRUE indicates pressure is within range"
    n158 = call "Wait Until Next Multiple8"("Count(mSec)"=u32 10 ("millisecond multiple")) -> ()  [unwired: 1 out]
    n159 = shared-variable "Trans-cRIO\\global trans shared var lib.lvlib\\Analyzer Image Interlock Bypass"() -> (w360:bool)  [unwired: 1 in, 1 out]
    n160 = shared-variable "Trans-cRIO\\global trans shared var lib.lvlib\\Switch Object Interlock Bypass"() -> (w359:bool)  [unwired: 1 in, 1 out]
    n161 = xnode "Read/Write Control"("FPGA VI Reference In"=w363, "Analyzer Image Interlock Bypass"=w360, "Switch Object Interlock Bypass"=w359) -> ("FPGA VI Reference Out"=w362:refnum<k20>, "error out"=w361:errorcluster)  [unwired: 1 in]
    n162 = xnode "Read/Write Control"("FPGA VI Reference In"=w362, "error in"=w361) -> ("error out"=w364:errorcluster, "Analyzer Image Vac Interlock"=w366:bool, "Switch Object Vac Interlock"=w365:bool)  [unwired: 1 out]
    "Interlock loop error" <- w364
    "Analyzer Image Vac Interlock" <- w366
    "Switch Object Vac Interlock" <- w365
    n163 = shared-variable "Trans-cRIO\\global trans shared var lib.lvlib\\Analyzer Image Vac Interlock"(w366) -> ()  [unwired: 1 in, 1 out]
    n164 = shared-variable ".\\local trans shared var lib.lvlib\\Interlock loop error"(w364) -> ()  [unwired: 1 in, 1 out]
    n165 = shared-variable "Trans-cRIO\\global trans shared var lib.lvlib\\Switch Object Vac Interlock"(w365) -> ()  [unwired: 1 in, 1 out]
  }
